vi "SwitchProc.vi"(8 "error in (no error)":errorcluster caption="entrée d'erreur (pas d'erreur)") -> (0 "error out":errorcluster caption="sortie d'erreur", 1 "Butée  +":bool[](array[boolean]), 2 "Butée -":bool[](array[boolean]))   [LabVIEW 2013]
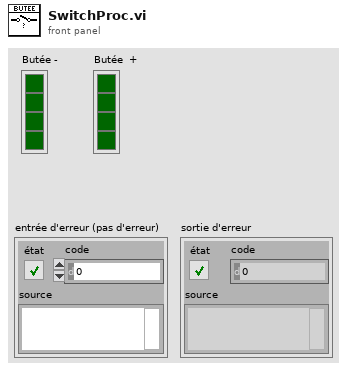
[diagram p1: front panel]
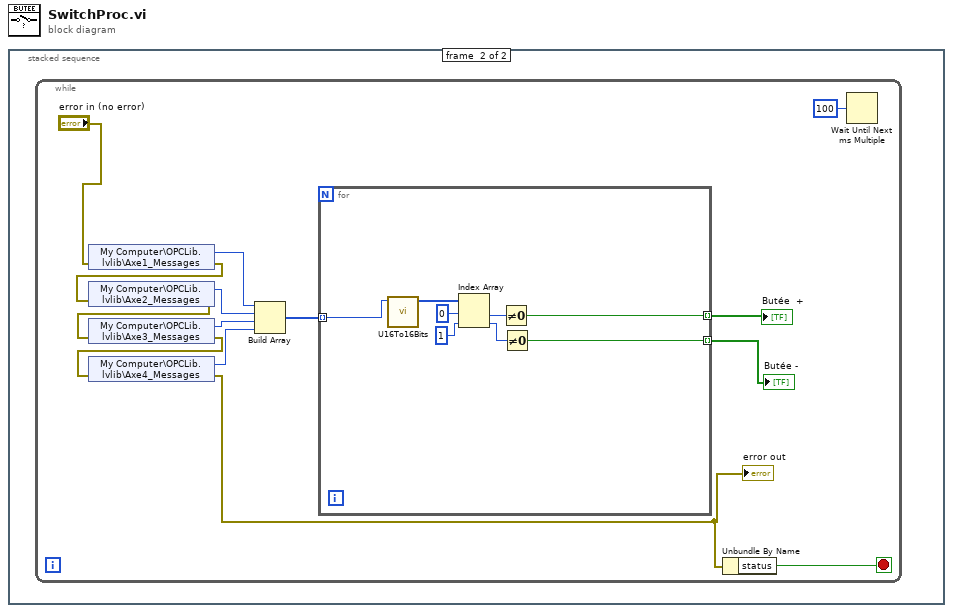
[diagram p0: block diagram]
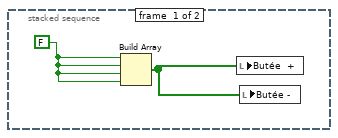
[diagram p2: hidden frame]
diagram:
  n1 = stacked-sequence {
    frame #0 {
      w2 = FALSE
      n2 = Build Array(w2, w2, w2, w2) -> (w1:bool[])
      n3 = local write "Butée  +"(w1) -> ()
      n4 = local write "Butée -"(w1) -> ()
    }
    frame #1 {
      n5 = while {
        stop <- w3 stop-if-true
        n6 = shared-variable "My Computer\\OPCLib.lvlib\\Axe1_Messages"(error in="error in (no error)") -> (w16:u16, error out=w8:errorcluster)
        n7 = shared-variable "My Computer\\OPCLib.lvlib\\Axe2_Messages"(error in=w8) -> (w15:u16, error out=w7:errorcluster)
        n8 = shared-variable "My Computer\\OPCLib.lvlib\\Axe3_Messages"(error in=w7) -> (w14:u16, error out=w6:errorcluster)
        n9 = shared-variable "My Computer\\OPCLib.lvlib\\Axe4_Messages"(error in=w6) -> (w13:u16, error out=w5:errorcluster)
        "error out" <- w5
        n10 = Build Array(w16, w15, w14, w13) -> (w12:u16[])
        n11 = for {
          tunnel: w12 -> [w19] mode=indexing
          tunnel: [w18] -> w11 mode=indexing
          tunnel: [w17] -> w10 mode=indexing
          n12 = call "U16To16Bits.vi"("Nombre à convertir"=w19) -> ("Array of bits"=w24:u16[])  [unwired: 10 in]
          n13 = Index Array(array=w24, index #1=0 ("index"), index #2=1 ("index")) -> (element #1=w21:u16, element #2=w20:u16)
          n14 = Not Equal To 0?(x=w21) -> (x != 0?=w18:bool)
          n15 = Not Equal To 0?(x=w20) -> (x != 0?=w17:bool)
        }
        "Butée  +" <- w11
        "Butée -" <- w10
        n16 = Unbundle By Name(w5) -> ("status"=w3:bool)
        n17 = Wait Until Next ms Multiple(millisecond multiple=u32 100 ("n millisecondes")) -> ()  [unwired: 1 out]
      }
    }
  }
